vi "subvi.vi"(8 "error in (no error)":errorcluster) -> (3 "Boolean":bool)   [LabVIEW 2020]
uses:
  <vilib>/measure/NI_MABase.lvlib
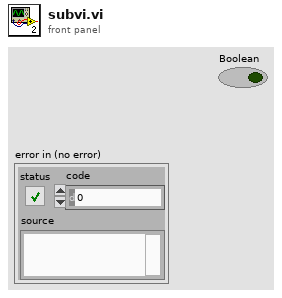
[diagram p1: front panel]
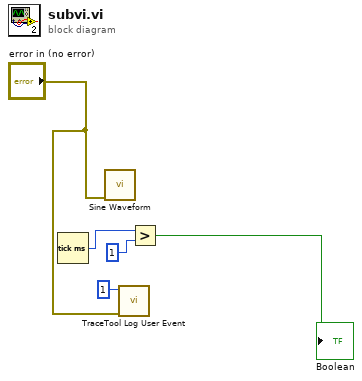
[diagram p0: block diagram]
diagram:
  n1 = Tick Count (ms)() -> (millisecond timer value=w1:u32)
  n2 = call <vilib>:"Sine Waveform.vi"("error in (no error)"="error in (no error)") -> ()  [unwired: 9 in, 2 out]
  n3 = call <vilib>:"TraceTool Log User Event.vi"("error in (no error)"="error in (no error)", "Event ID (0-255)"=u32 1) -> ()  [unwired: 9 in, 1 out]
  n4 = Greater?(x=w1, y=u32 1) -> (0:→"Boolean":bool)
